vi "isTdc.vi"(8 "error in (no error)":errorcluster) -> (0 "error out":errorcluster, 2 "isTdc2":bool, 3 "isTdc1":bool)   [LabVIEW 2015, in "ESLSCDLL.lvlib"]
uses:
  ESLSCDLL.lvlib
  Globals.vi
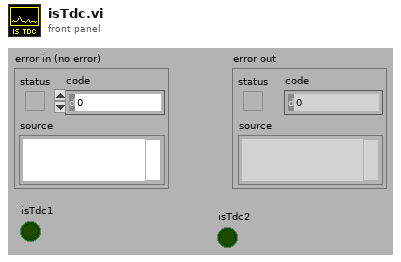
[diagram p1: front panel]
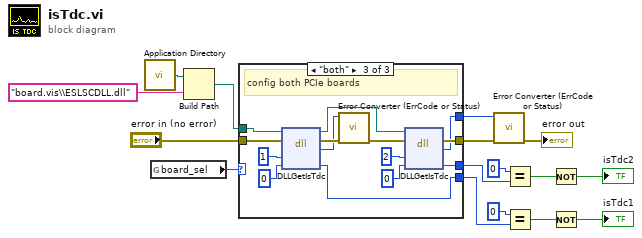
[diagram p0: block diagram]
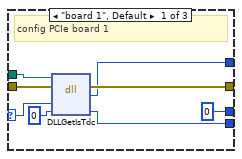
[diagram p2: hidden frame]
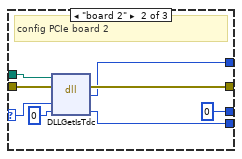
[diagram p3: hidden frame]
diagram:
  n1 = call <vilib>:"Application Directory.vi"() -> ("Application Directory"=w3:path)
  n2 = global read "Globals.vi" "board_sel"() -> (w4:enum32{"0", "board 1", "board 2", "both"})
  n3 = Build Path(base path=w3, name or relative path="board.vis\\ESLSCDLL.dll") -> (appended path=w1:path)
  n4 = case shown="\"both\"" w4 {
    selector: w4 -> [w23 w31 _]
    tunnel: [w19 w28 w36] -> w13
    tunnel: [u8 0 ("BlockOn") u8 0 ("BlockOn") w35] -> w10
    tunnel: "error in (no error)" -> [w22 w30 w42]
    tunnel: [w21 w27 w38] -> w6
    tunnel: [w18 w26 w37] -> w5
    tunnel: w1 -> [w17 w25 w34]
    frame "board 1", Default {
      # "config PCIe board 1"
      n5 = dll-call lib="C:/ENTW/PCIE/LV64/board.vis/ESLSCDLL.dll" fn="DLLGetIsTdc" ("lwlscdll.dll:DLLWriteLongS0")(path in=w17, error in=w22, "drv"=w23, "isTdc"=u8 0 ("measureOn")) -> (error out=w21:errorcluster, "es_status_codes"=w18:i32, "isTdc"=w19:u8)  [unwired: 2 in, 1 out]
    }
    frame "board 2" {
      # "config PCIe board 2"
      n6 = dll-call lib="C:/ENTW/PCIE/LV64/board.vis/ESLSCDLL.dll" fn="DLLGetIsTdc" ("lwlscdll.dll:DLLWriteLongS0")(path in=w25, error in=w30, "drv"=w31, "isTdc"=u8 0 ("measureOn")) -> (error out=w27:errorcluster, "es_status_codes"=w26:i32, "isTdc"=w28:u8)  [unwired: 2 in, 1 out]
    }
    frame "both" {
      # "config both PCIe boards"
      n7 = dll-call lib="C:/ENTW/PCIE/LV64/board.vis/ESLSCDLL.dll" fn="DLLGetIsTdc" ("lwlscdll.dll:DLLWriteLongS0")(path in=w34, error in=w42, "drv"=u32 1, "isTdc"=u8 0 ("measureOn")) -> (path out=w33:path, error out=w41:errorcluster, "es_status_codes"=w40:i32, "isTdc"=w36:u8)  [unwired: 2 in]
      n8 = call "Error Converter (ErrCode or Status).vi"("error in (no error)"=w41, "error code"=w40) -> ("error out"=w39:errorcluster)  [unwired: 9 in]
      n9 = dll-call lib="C:/ENTW/PCIE/LV64/board.vis/ESLSCDLL.dll" fn="DLLGetIsTdc" ("lwlscdll.dll:DLLWriteLongS0")(path in=w33, error in=w39, "drv"=u32 2, "isTdc"=u8 0 ("measureOn")) -> (error out=w38:errorcluster, "es_status_codes"=w37:i32, "isTdc"=w35:u8)  [unwired: 2 in, 1 out]
    }
  }
  n10 = call "Error Converter (ErrCode or Status).vi"("error in (no error)"=w6, "error code"=w5) -> ("error out"=→"error out":errorcluster)  [unwired: 9 in]
  n11 = Equal?(x=u8 0, y=w10) -> (x = y?=w11:bool)
  n12 = Equal?(x=u8 0, y=w13) -> (x = y?=w15:bool)
  n13 = Not(x=w11) -> (.not. x?=→"isTdc2":bool)
  n14 = Not(x=w15) -> (.not. x?=→"isTdc1":bool)
